vi "Test XYZ Table Stage Module All Axis.vi"() -> ()   [LabVIEW 2014]
uses:
  Hardware/Table Stage/Controls/Translation Stage Cluster.ctl
  General/Controls/Translation Stage Types.ctl
  General/Controls/Set Get Controls.ctl
  Hardware/Table Stage/Controls/Motion Translation Module Control.ctl
panel:
  out "Cluster":T3
  in  "Z Pos":dbl caption="Position"
  in  "Y Pos":dbl caption="Position"
  in  "X Pos":dbl caption="Position"
  out "Error Out":errorcluster
  in  "Uninit":bool
  in  "Init":bool
  in  "Cancel Button":bool
  in  "Position":bool
  in  "Stop":bool
  in  "Home":bool
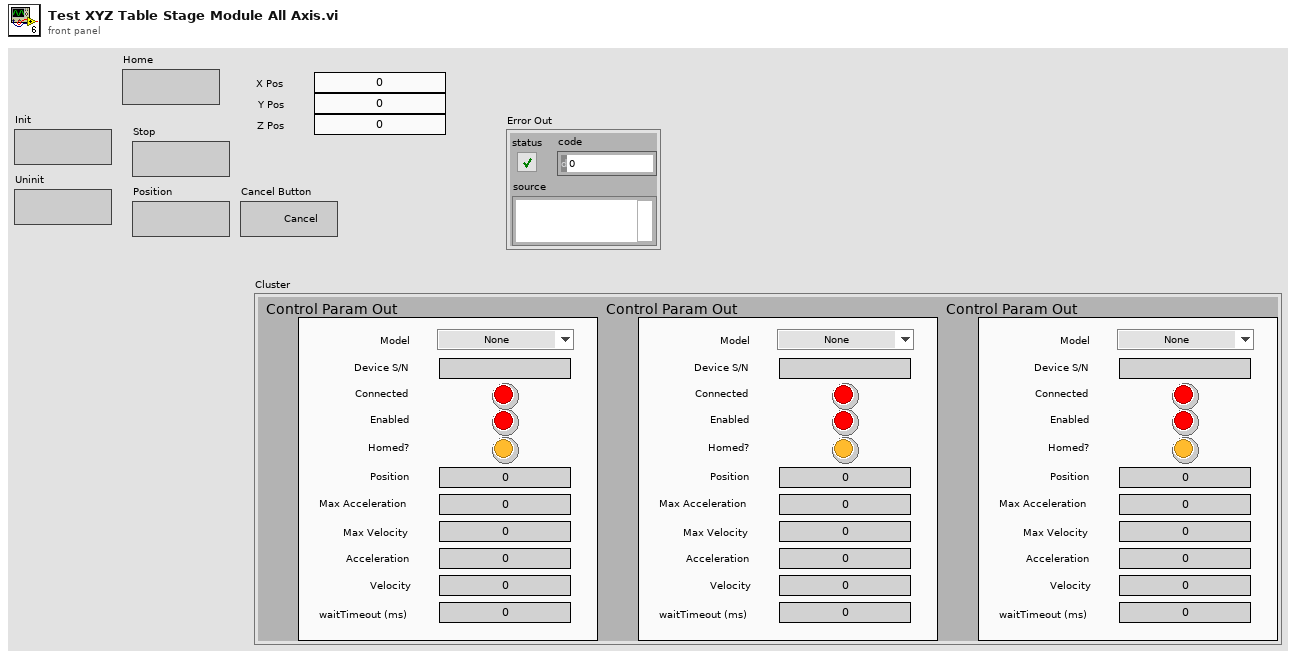
[diagram p1: front panel]
types:
  T1 = typedef "Translation Stage Cluster.ctl" = cluster{"Position":dbl, "Is.Enabled?":bool, "Is.Connected?":bool, "Device SN":string, "AccelerationMaximum":dbl, "VelocityMaximum":dbl, "Acceleration":dbl, "Velocity":dbl, "waitTimeout (ms)":i32, "Model":T2, "Is.Homed?":bool}
  T2 = typedef "Translation Stage Types.ctl" = enum16{"None", "Thorlabs LTS", "Thorlabs MLJ"}
  T3 = cluster{"Control Param Out":T1, "Control Param Out":T1, "Control Param Out":T1}
  T4 = typedef "Motion Translation Module Control.ctl" = enum16{"Init", "Home", "Status", "Velocity/Accel", "Position", "Jog", "Stop", "Uninit", "Enable", "Disable"}
  T5 = typedef "Set Get Controls.ctl" = enum16{"Set", "Get"}
  T6 = cluster{"X Stage":T1, "Y Stage":T1, "Z Stage":T1}
  T7 = typedef "System Parameters.ctl" = cluster{"OCT":cluster{"Focal Length":dbl[unit]}, "Vibratome":cluster{"Z Bottom [mm]":dbl, "Pre Cut Dwell [s]":dbl, "Blade Frequency [RPM]":u16, "Slice Speed [mm/s]":dbl, "Post Cut Dwell [s]":dbl, "Ramp Time [s]":dbl, "Start X [mm]":dbl, "Start Y [mm]":dbl, "Slice Length [mm]":dbl, "Slice Axis":enum16{"X Axis", "Y Axis", "Z Axis"}, "Controller VISA Ref":refnum<visa-resource-name>}, "Table Stages":cluster{"X Stage":T1, "Y Stage":T1, "Z Stage":T1}}
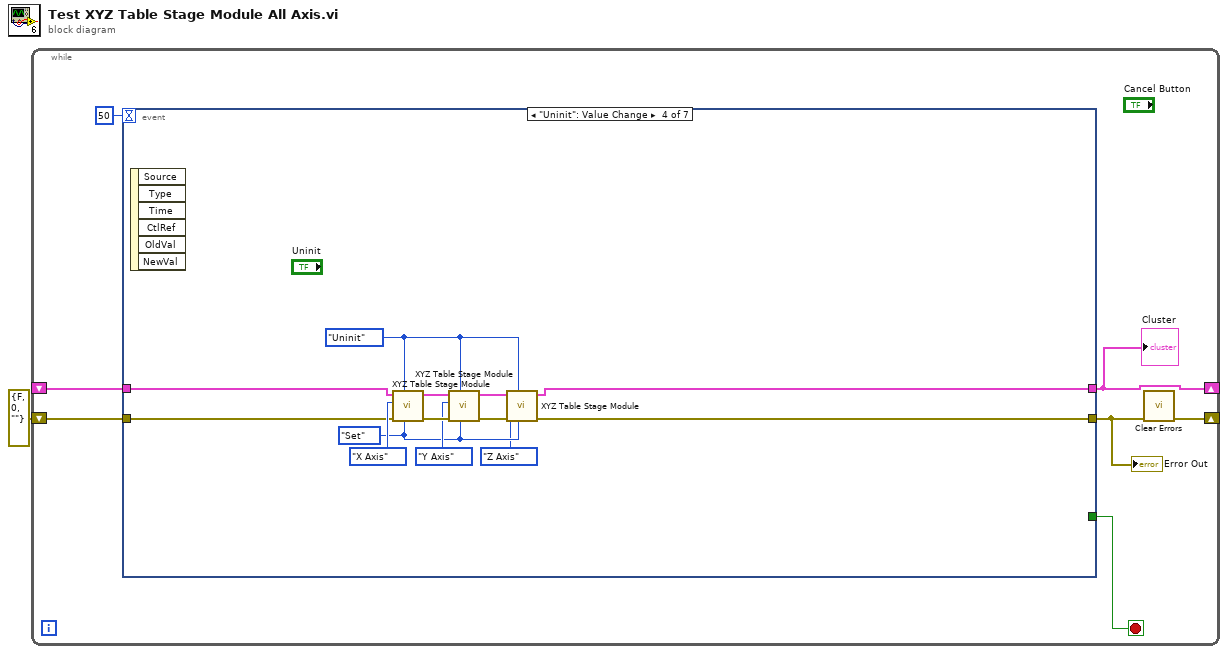
[diagram p0: block diagram]
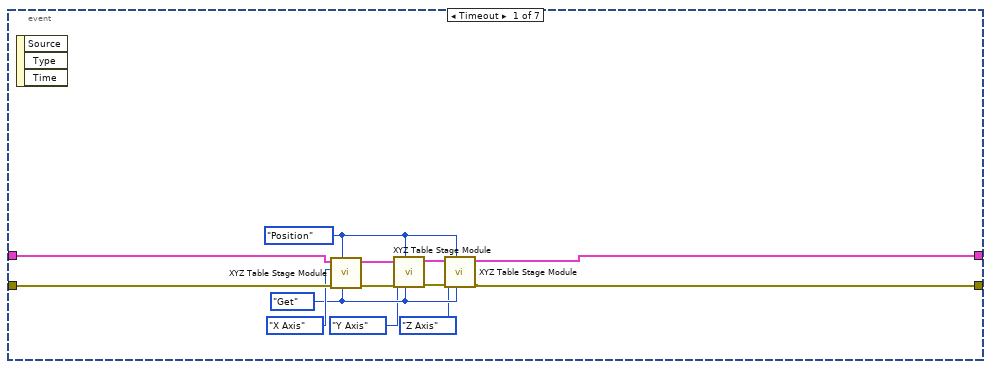
[diagram p2: hidden frame]
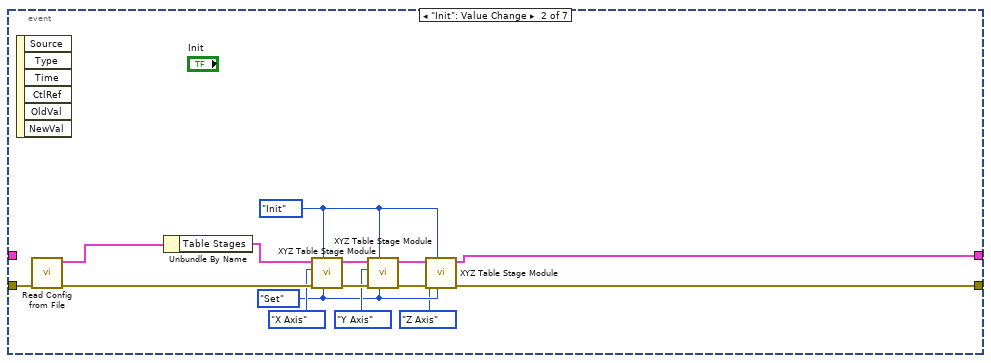
[diagram p3: hidden frame]
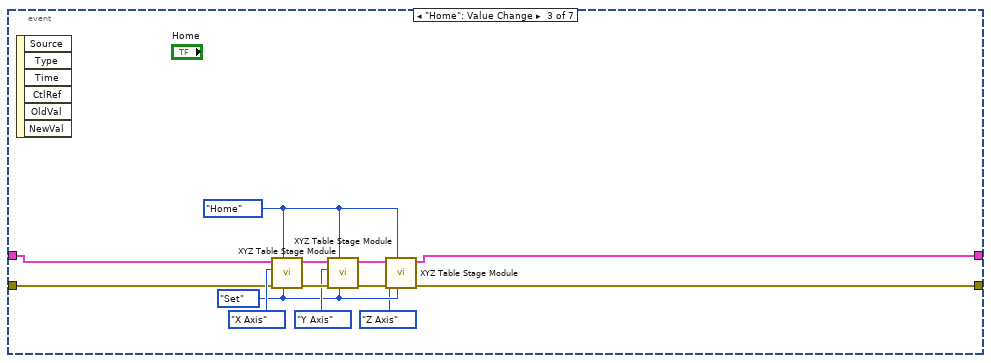
[diagram p4: hidden frame]
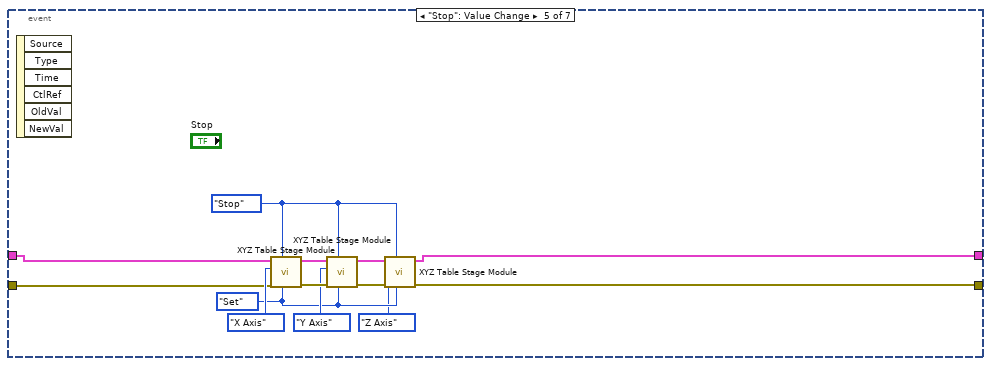
[diagram p5: hidden frame]
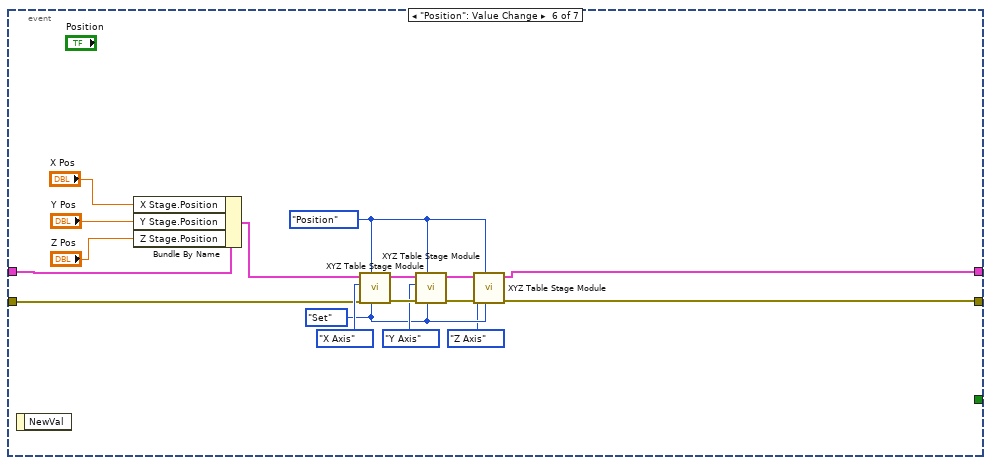
[diagram p6: hidden frame]
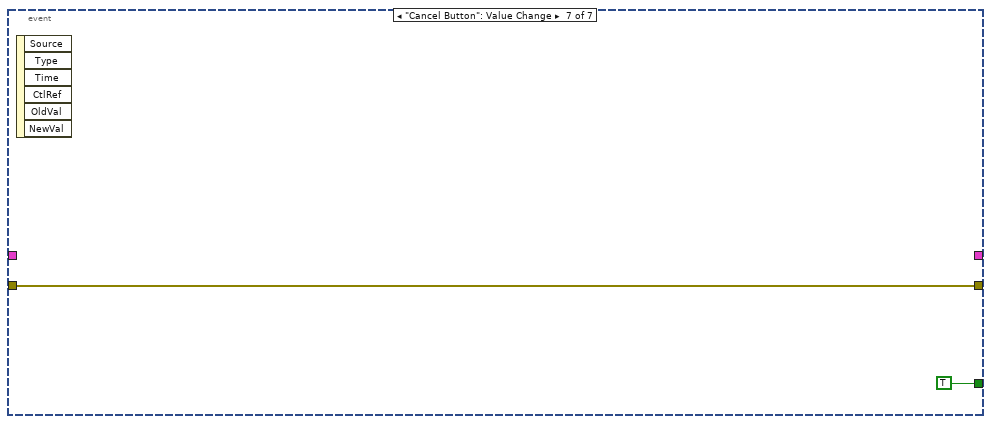
[diagram p7: hidden frame]
diagram:
  n1 = while {
    shift-right: [w3] -> _
    shift-left: errorcluster {"status"=FALSE, "code"=0, "source"=""} ("Error Out") -> [w5]
    shift-right: [w2] -> _
    shift-left: _ -> [w4]
    stop <- w7 stop-if-true
    n2 = event shown="[3] \"Uninit\": Value Change" {
      selector: _ -> [_ _ _ _ _ _ _]
      dyn-events: _ -> [_ _ _ _ _ _ _]
      timeout: 50 -> [_ _ _ _ _ _ _]
      tunnel: [_ _ _ _ _ _ TRUE] -> w7
      tunnel: [w9 w22 w37 w50 w63 w76 _] -> w2
      tunnel: w4 -> [w20 _ w40 w53 w66 w80 _]
      tunnel: [w10 w32 w41 w54 w67 w83 w93] -> w6
      tunnel: w5 -> [w21 w35 w42 w55 w68 w84 w93]
      event Timeout {
        w14 = Motion_Translation_Module_Control."Position" ("Action")
        w13 = Set_Get_Controls."Get" ("Set/Get")
        n3 = event-data() -> ()  [unwired: 1 in, 3 out]
        n4 = call "XYZ Table Stage Module.vi"("Set/Get"=w13, "Action"=w14, "Error In"=w21, "Axis"=enum16{"X Axis", "Y Axis", "Z Axis"}."X Axis", "Table Stages"=w20) -> ("Error Out"=w16:errorcluster, "Table Stages Out"=w15:T6)  [unwired: 5 in]
        n5 = call "XYZ Table Stage Module.vi"("Set/Get"=w13, "Action"=w14, "Error In"=w16, "Axis"=enum16{"X Axis", "Y Axis", "Z Axis"}."Y Axis", "Table Stages"=w15) -> ("Error Out"=w18:errorcluster, "Table Stages Out"=w17:T6)  [unwired: 5 in]
        n6 = call "XYZ Table Stage Module.vi"("Set/Get"=w13, "Action"=w14, "Error In"=w18, "Axis"=enum16{"X Axis", "Y Axis", "Z Axis"}."Z Axis", "Table Stages"=w17) -> ("Error Out"=w10:errorcluster, "Table Stages Out"=w9:T6)  [unwired: 5 in]
      }
      event "Init": Value Change {
        w28 = Set_Get_Controls."Set" ("Set/Get")
        w26 = Motion_Translation_Module_Control."Init" ("Action")
        n7 = event-data() -> ()  [unwired: 1 in, 6 out]
        n8 = call "Read Config from File.vi"("error in (no error)"=w35) -> ("error out"=w34:errorcluster, "System Parameters"=w31:T7)  [unwired: 9 in]
        n9 = Unbundle By Name(w31) -> ("Table Stages"=w25:T6)
        n10 = call "XYZ Table Stage Module.vi"("Set/Get"=w28, "Action"=w26, "Error In"=w34, "Axis"=enum16{"X Axis", "Y Axis", "Z Axis"}."X Axis", "Table Stages"=w25) -> ("Error Out"=w33:errorcluster, "Table Stages Out"=w24:T6)  [unwired: 5 in]
        n11 = call "XYZ Table Stage Module.vi"("Set/Get"=w28, "Action"=w26, "Error In"=w33, "Axis"=enum16{"X Axis", "Y Axis", "Z Axis"}."Y Axis", "Table Stages"=w24) -> ("Error Out"=w36:errorcluster, "Table Stages Out"=w23:T6)  [unwired: 5 in]
        n12 = call "XYZ Table Stage Module.vi"("Set/Get"=w28, "Action"=w26, "Error In"=w36, "Axis"=enum16{"X Axis", "Y Axis", "Z Axis"}."Z Axis", "Table Stages"=w23) -> ("Error Out"=w32:errorcluster, "Table Stages Out"=w22:T6)  [unwired: 5 in]
      }
      event "Home": Value Change {
        w45 = Set_Get_Controls."Set" ("Set/Get")
        w43 = Motion_Translation_Module_Control."Home" ("Action")
        n13 = event-data() -> ()  [unwired: 1 in, 6 out]
        n14 = call "XYZ Table Stage Module.vi"("Set/Get"=w45, "Action"=w43, "Error In"=w42, "Axis"=enum16{"X Axis", "Y Axis", "Z Axis"}."X Axis", "Table Stages"=w40) -> ("Error Out"=w48:errorcluster, "Table Stages Out"=w39:T6)  [unwired: 5 in]
        n15 = call "XYZ Table Stage Module.vi"("Set/Get"=w45, "Action"=w43, "Error In"=w48, "Axis"=enum16{"X Axis", "Y Axis", "Z Axis"}."Y Axis", "Table Stages"=w39) -> ("Error Out"=w49:errorcluster, "Table Stages Out"=w38:T6)  [unwired: 5 in]
        n16 = call "XYZ Table Stage Module.vi"("Set/Get"=w45, "Action"=w43, "Error In"=w49, "Axis"=enum16{"X Axis", "Y Axis", "Z Axis"}."Z Axis", "Table Stages"=w38) -> ("Error Out"=w41:errorcluster, "Table Stages Out"=w37:T6)  [unwired: 5 in]
      }
      event "Uninit": Value Change {
        w58 = Set_Get_Controls."Set" ("Set/Get")
        w56 = Motion_Translation_Module_Control."Uninit" ("Action")
        n17 = event-data() -> ()  [unwired: 1 in, 6 out]
        n18 = call "XYZ Table Stage Module.vi"("Set/Get"=w58, "Action"=w56, "Error In"=w55, "Axis"=enum16{"X Axis", "Y Axis", "Z Axis"}."X Axis", "Table Stages"=w53) -> ("Error Out"=w61:errorcluster, "Table Stages Out"=w52:T6)  [unwired: 5 in]
        n19 = call "XYZ Table Stage Module.vi"("Set/Get"=w58, "Action"=w56, "Error In"=w61, "Axis"=enum16{"X Axis", "Y Axis", "Z Axis"}."Y Axis", "Table Stages"=w52) -> ("Error Out"=w62:errorcluster, "Table Stages Out"=w51:T6)  [unwired: 5 in]
        n20 = call "XYZ Table Stage Module.vi"("Set/Get"=w58, "Action"=w56, "Error In"=w62, "Axis"=enum16{"X Axis", "Y Axis", "Z Axis"}."Z Axis", "Table Stages"=w51) -> ("Error Out"=w54:errorcluster, "Table Stages Out"=w50:T6)  [unwired: 5 in]
      }
      event "Stop": Value Change {
        w71 = Set_Get_Controls."Set" ("Set/Get")
        w69 = Motion_Translation_Module_Control."Stop" ("Action")
        n21 = event-data() -> ()  [unwired: 1 in, 6 out]
        n22 = call "XYZ Table Stage Module.vi"("Set/Get"=w71, "Action"=w69, "Error In"=w68, "Axis"=enum16{"X Axis", "Y Axis", "Z Axis"}."X Axis", "Table Stages"=w66) -> ("Error Out"=w74:errorcluster, "Table Stages Out"=w65:T6)  [unwired: 5 in]
        n23 = call "XYZ Table Stage Module.vi"("Set/Get"=w71, "Action"=w69, "Error In"=w74, "Axis"=enum16{"X Axis", "Y Axis", "Z Axis"}."Y Axis", "Table Stages"=w65) -> ("Error Out"=w75:errorcluster, "Table Stages Out"=w64:T6)  [unwired: 5 in]
        n24 = call "XYZ Table Stage Module.vi"("Set/Get"=w71, "Action"=w69, "Error In"=w75, "Axis"=enum16{"X Axis", "Y Axis", "Z Axis"}."Z Axis", "Table Stages"=w64) -> ("Error Out"=w67:errorcluster, "Table Stages Out"=w63:T6)  [unwired: 5 in]
      }
      event "Position": Value Change {
        w87 = Set_Get_Controls."Set" ("Set/Get")
        w85 = Motion_Translation_Module_Control."Position" ("Action")
        n25 = event-data() -> ()  [unwired: 1 in, 1 out]
        n26 = Bundle By Name(cluster=w80, "X Stage.Position"="X Pos", "Y Stage.Position"="Y Pos", "Z Stage.Position"="Z Pos") -> (w79:T6)
        n27 = call "XYZ Table Stage Module.vi"("Set/Get"=w87, "Action"=w85, "Error In"=w84, "Axis"=enum16{"X Axis", "Y Axis", "Z Axis"}."X Axis", "Table Stages"=w79) -> ("Error Out"=w90:errorcluster, "Table Stages Out"=w78:T6)  [unwired: 5 in]
        n28 = call "XYZ Table Stage Module.vi"("Set/Get"=w87, "Action"=w85, "Error In"=w90, "Axis"=enum16{"X Axis", "Y Axis", "Z Axis"}."Y Axis", "Table Stages"=w78) -> ("Error Out"=w91:errorcluster, "Table Stages Out"=w77:T6)  [unwired: 5 in]
        n29 = call "XYZ Table Stage Module.vi"("Set/Get"=w87, "Action"=w85, "Error In"=w91, "Axis"=enum16{"X Axis", "Y Axis", "Z Axis"}."Z Axis", "Table Stages"=w77) -> ("Error Out"=w83:errorcluster, "Table Stages Out"=w76:T6)  [unwired: 5 in]
      }
      event "Cancel Button": Value Change {
        n30 = event-data() -> ()  [unwired: 1 in, 6 out]
      }
    }
    "Error Out" <- w6
    "Cluster" <- w2
    n31 = call <vilib>:"Clear Errors.vi"("error in (no error)"=w6) -> ("error out"=w3:errorcluster)  [unwired: 5 in, 1 out]
  }
